vi "X1 Encoder Count.vi"(4 "phase B_prev":bool, 5 "phase A":bool, 6 "phase B":bool, 7 "phase A_prev":bool, 11 "count in":i32) -> (2 "count changed?":bool, 3 "count out":i32)   [LabVIEW 2017, in "NI_Robotics Utilities.lvlib"]
uses:
  <vilib>/robotics/Utilities/NI_Robotics Utilities.lvlib
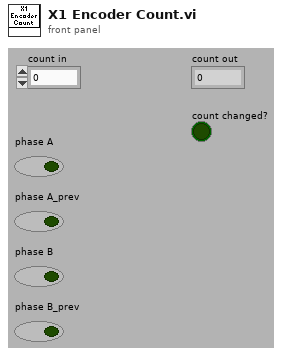
[diagram p1: front panel]
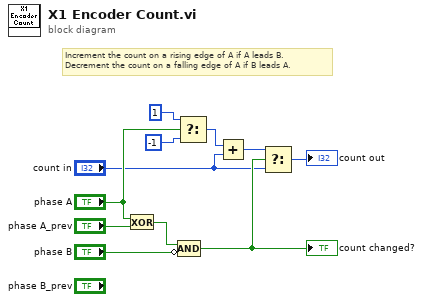
[diagram p0: block diagram]
diagram:
  # "Increment the count on a rising edge of A if A leads B.\nDecrement the count on a falling edge of A if B leads A."
  n1 = Exclusive Or(1:"phase A_prev", 2:"phase A") -> (0:w9:bool)
  n2 = Select(t=1 ("count in"), s="phase A", f=-1 ("count in")) -> (s? t:f=w2:i32)
  n3 = Compound Arithmetic op=AND(w9, invert "phase B") -> (w7:bool)
  "count changed?" <- w7
  n4 = Add(x=w2, y="count in") -> (x+y=w1:i32)
  n5 = Select(t=w1, s=w7, f="count in") -> (s? t:f=→"count out":i32)
